vi "MTMount_getEvent_axesInPosition.vi"(8 "error in (no error)":errorcluster, 11 "logevent_axesInPosition_Ctl":T1) -> (0 "error out":errorcluster, 2 "function return":i32, 3 "logevent_axesInPosition_Ctl out":T1)   [LabVIEW 2018, in "SALLV_MTMount.lvlib"]
doc: "int MTMount_shm_getEvent_axesInPositionLV(MTMount_logevent_axesInPositionLV *logevent_axesInPosition_Ctl );"
uses:
  DataTypes/logevent_axesInPosition.ctl
  SALLV_MTMount.lvlib
  SALLV_MTMount.so
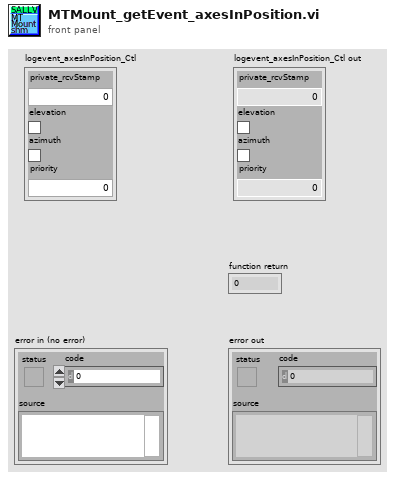
[diagram p1: front panel]
types:
  T1 = typedef "SALLV_MTMount.lvlib/logevent_axesInPosition.ctl" = cluster{"private_rcvStamp":dbl, "elevation":bool, "azimuth":bool, "priority":i32}
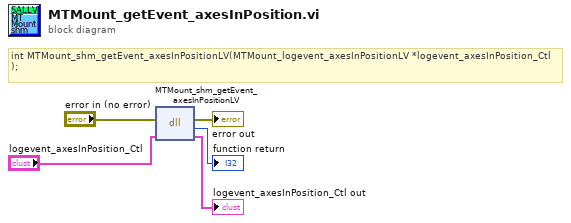
[diagram p0: block diagram]
diagram:
  # "int MTMount_shm_getEvent_axesInPositionLV(MTMount_logevent_axesInPositionLV *logevent_axesInPosition_Ctl );"
  n1 = dll-call lib="home/ttsai/Documents/salLabviewApi/SALLV_MTMount/SALLV_MTMount.*" fn="MTMount_shm_getEvent_axesInPositionLV"(error in="error in (no error)", "logevent_axesInPosition_Ctl"="logevent_axesInPosition_Ctl") -> (error out=→"error out":errorcluster, →"function return":i32, "logevent_axesInPosition_Ctl"=→"logevent_axesInPosition_Ctl out":T1)  [unwired: 2 in, 1 out]
